vi "Producer Consumer Template.vi"() -> ()   [LabVIEW 2021]
uses:
  <vilib>/platform/TimedLoop/XDataNode/XDataNode.xnode
  <vilib>/Platform/TimedLoop/XDataNode/nitl_modes.ctl
  <vilib>/Platform/TimedLoop/XDataNode/XDNodeRunTimeDep.lvlib
  <vilib>/Platform/TimedLoop/XDataNode/wakeup.ctl
  <vilib>/Platform/TimedLoop/XDataNode/timing_clust.ctl
panel:
  in  "stop":bool
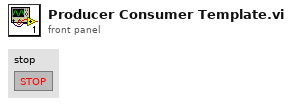
[diagram p1: front panel]
types:
  T1 = typedef "XDNodeRunTimeDep.lvlib/timing_clust.ctl" = cluster{"Expected End [f-1]":u64, "Actual End [f-1]":u64, "Finished Late? [f-1]":bool, "Expected End [i-1]":u64, "Actual End [i-1]":u64, "Finished Late? [i-1]":bool, "Expected Start [i]":u64, "Actual Start [i]":u64, "Expected Start [f]":u64, "Actual Start [f]":u64, "Source Name":string, "Structure Name":string, "Period":i64, "Deadline":i64, "Offset":i64, "Start":i64, "Priority":i32, "Timeout":i32, "Mode":T2, "Wakeup Reason":T3, "Error":errorcluster, "Source Type":string, "Secondary Source Type":string, "Global End Time":u64, "Global Start Time":u64, "Frame Duration":u64, "Iteration Duration":u64, "Assigned CPU":i32, "I/O Scan Engine Mode":u32}
  T2 = typedef "XDNodeRunTimeDep.lvlib/nitl_modes.ctl" = enum32{"No Change", "Process missed periods, maintain original phase", "Discard missed periods, maintain original phase", "Process missed periods, ignore original phase", "Discard missed periods, ignore original phase"}
  T3 = typedef "XDNodeRunTimeDep.lvlib/wakeup.ctl" = enum32{"Normal", "Aborted", "Asynchronous wakeup", "Timing source error", "Timed loop error", "Timeout"}
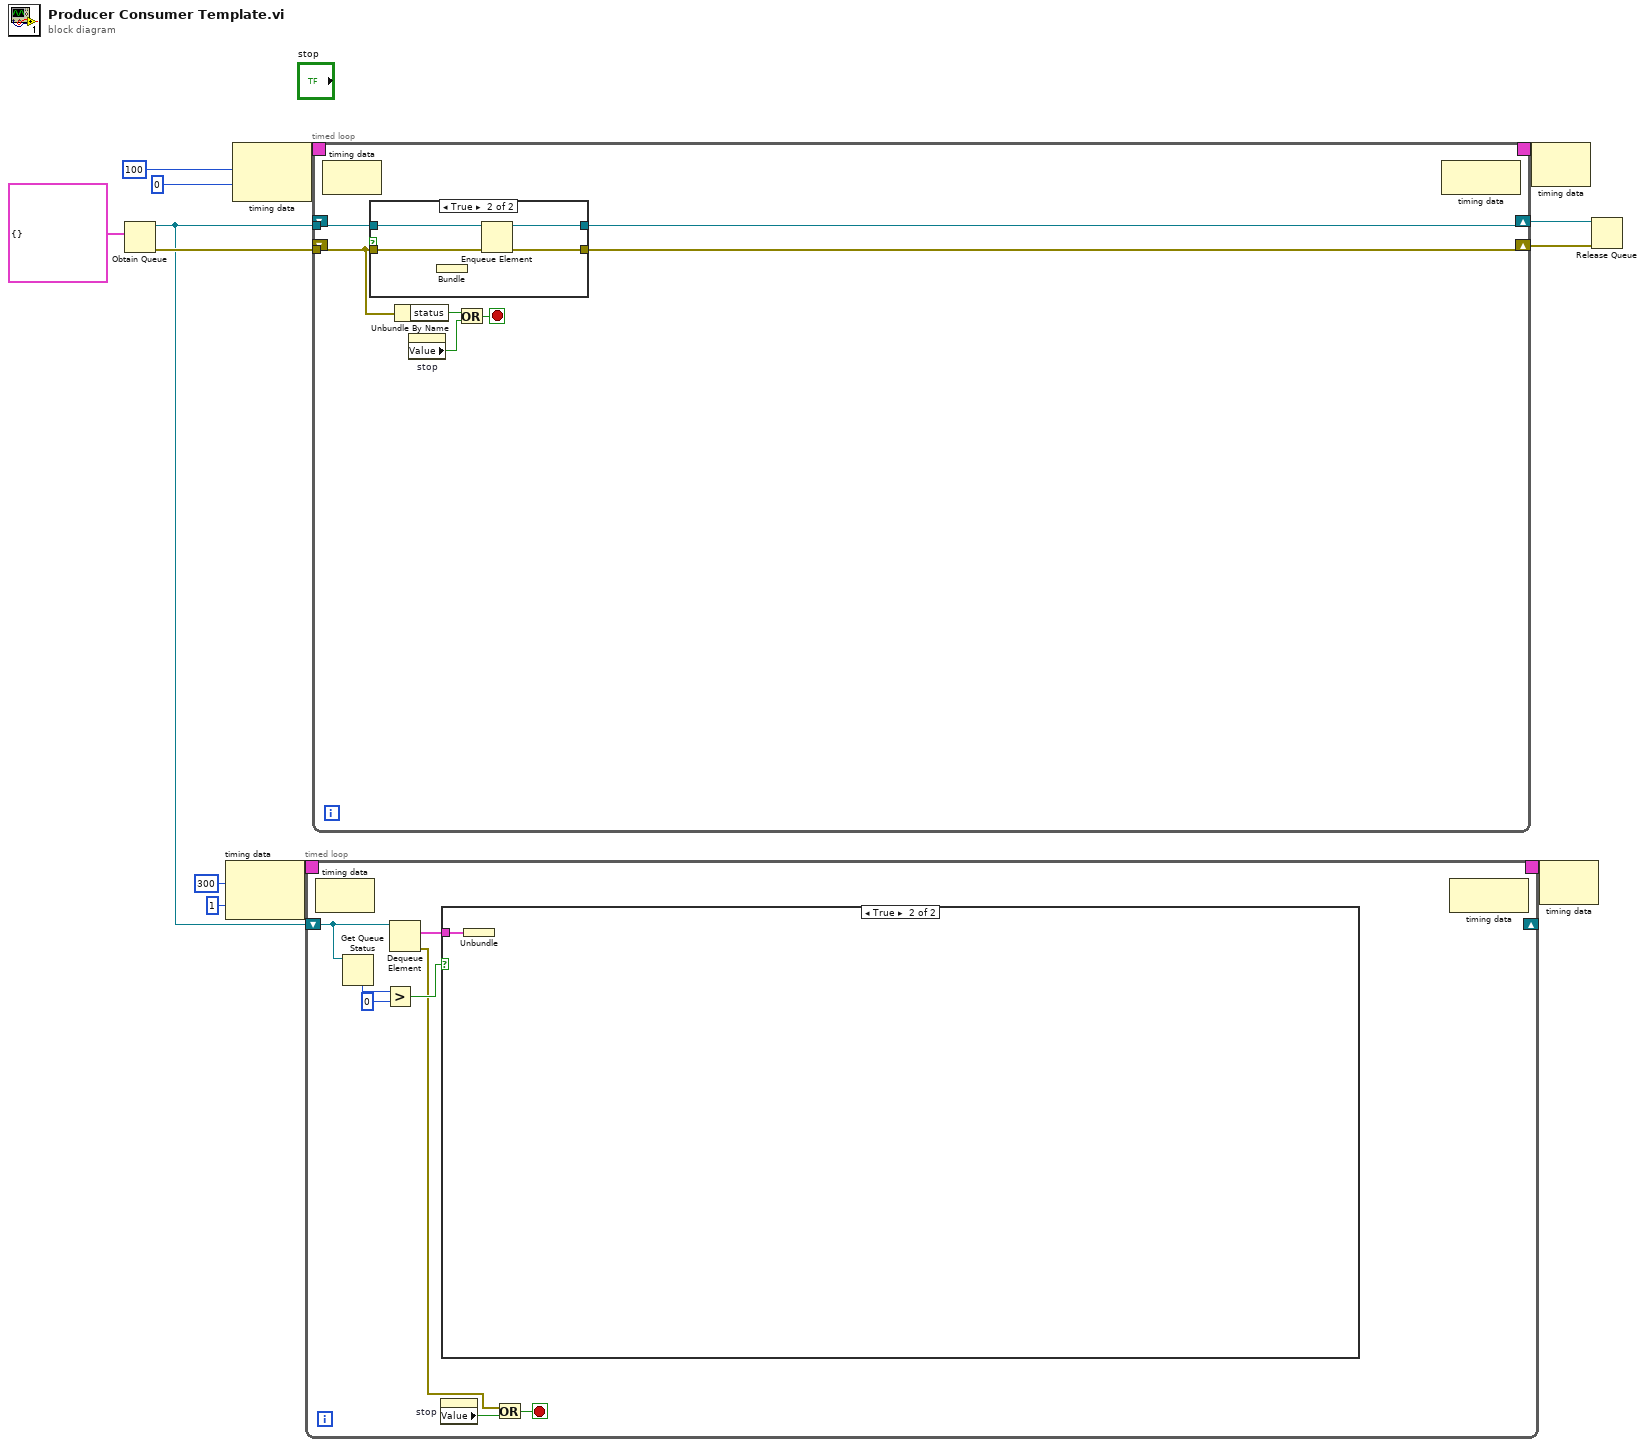
[diagram p0: block diagram]
diagram:
  n1 = Obtain Queue(element data type=cluster{} {}) -> (queue out=w5:refnum<queue>, error out=w6:errorcluster)  [unwired: 4 in, 1 out]
  n2 = node-c288(i64 300 ("Period"), 1 ("Processor")) -> (w11:T1)
  n3 = node-c288(i64 100 ("Period"), 0 ("Processor")) -> (w13:T1)
  n4 = timed-loop {
    timing: w11 -> [_]
    timing-out: [_] -> w10
    shift-right: _ -> [_]
    shift-left: w5 -> [w18]
    stop <- w16 stop-if-true
    n5 = node-c288() -> ()  [unwired: 1 in, 1 out]
    n6 = Get Queue Status(queue=w18) -> (# elements in queue=w19:i32)  [unwired: 2 in, 7 out]
    n7 = Greater?(x=w19, y=0) -> (0:w17:bool)
    n8 = Dequeue Element(queue=w18) -> (element=w21:cluster{}, error out=w14:errorcluster)  [unwired: 2 in, 2 out]
    n9 = property on="stop" class="Bool (strict)"() -> ("Value"=w15:bool)  [unwired: 2 in, 2 out]
    n10 = case shown="True" w17 {
      tunnel: w21 -> [_ w22]
      frame False {
      }
      frame True {
        n11 = Unbundle(w22) -> ()  [unwired: 1 out]
      }
    }
    n12 = Or(x=w14, y=w15) -> (x .or. y?=w16:bool)
    n13 = node-c288() -> ()  [unwired: 1 in, 1 out]
  }
  n14 = timed-loop {
    timing: w13 -> [_]
    timing-out: [_] -> w12
    tunnel: w5 -> [w31]
    tunnel: w6 -> [w27]
    shift-right: [w30] -> w4
    shift-left: _ -> [_]
    shift-right: [w28] -> w2
    shift-left: _ -> [_]
    stop <- w29 stop-if-true
    n15 = node-c288() -> ()  [unwired: 1 in, 1 out]
    n16 = case shown="True" {
      selector: _ -> [_ _]
      tunnel: w31 -> [w33 w37]
      tunnel: w27 -> [w32 w36]
      tunnel: [w32 w35] -> w30
      tunnel: [w33 w34] -> w28
      frame False {
      }
      frame True {
        n17 = Bundle() -> ()  [unwired: 2 in, 1 out]
        n18 = Enqueue Element(queue=w37, error in (no error)=w36) -> (queue out=w34:refnum<queue>, error out=w35:errorcluster)  [unwired: 2 in, 1 out]
      }
    }
    n19 = Unbundle By Name(w27) -> ("status"=w26:bool)
    n20 = property on="stop" class="Bool (strict)"() -> ("Value"=w25:bool)  [unwired: 2 in, 2 out]
    n21 = Or(x=w26, y=w25) -> (x .or. y?=w29:bool)
    n22 = node-c288() -> ()  [unwired: 1 in, 1 out]
  }
  n23 = node-c288(w12) -> ()  [unwired: 1 out]
  n24 = node-c288(w10) -> ()  [unwired: 1 out]
  n25 = Release Queue(queue=w2, error in (no error)=w4) -> ()  [unwired: 1 in, 3 out]
